vi "LV to ITX AutoPlot.vi"(0 "filename":string="filename", 1 "path":path=path "C:/", 5 "Notes":string, 7 "Data":cluster{"Y  Array":dbl[]}[](array[cluster]), 11 "wavenames (.Vx, etc)":string[](array[string])=["time", "x", "y", "z"], 12 "X,Y Labels":string[](array[string])=["x label", "y label"], 13 "X,Y Log":i32[](array[numeric])) -> (4 "file":path)   [LabVIEW 2013]
doc: "Write data to ITX file. This AutoPlot VI adds commands to automatically create a graph in Igor to quickly view your data.\n\n-- path: base path to save data\n-- filename: base filename\n-- Notes: add any notes here to help you remember what experiment you did\n-- Data: Cluster array\n It is recommended that you make the first cluster an array of timestamps\n-- wavenames: Give each data array a unique name such as \"time, bias, current,...\"zz\n-- X,Y Labels: For plotting in Igor. Can be ignored.\n-- X,Y Log: Do you wan to show X or Y on Log scale in Igor?"
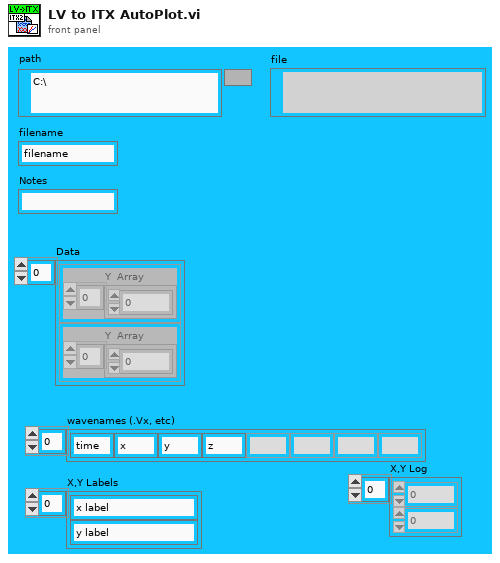
[diagram p1: front panel]
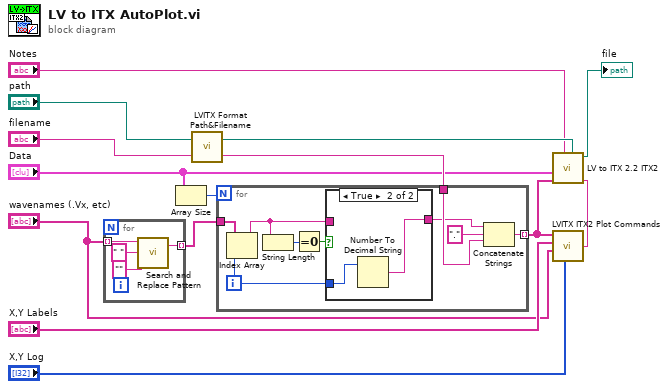
[diagram p0: block diagram]
diagram:
  n1 = for {
    tunnel: "wavenames (.Vx, etc)" -> [w16] mode=indexing
    tunnel: [w15] -> w1 mode=indexing
    n2 = call <vilib>:"Search and Replace Pattern.vi"("string"=w16, "regular expression (\"\")"=" " ("regular expression (\"\")"), "replace string (\"\")"="" ("replace string (\"\")")) -> ("result string"=w15:string)  [unwired: 2 in, 1 out]
  }
  n3 = Array Size(array="Data") -> (size(s)=w13:i32)
  n4 = call "LVITX Format Path&Filename.vi"("filename"="filename", "path"="path") -> ("file name without extension"=w12:string, "dup file"=w9:path)
  n5 = for {
    N: w13 -> [_]
    tunnel: w1 -> [w22]
    tunnel: w12 -> [w20]
    tunnel: [w27] -> w2 mode=indexing
    i -> [w23]
    n6 = Index Array(array=w22, index=w23) -> (element=w21:string)
    n7 = String Length(string=w21) -> (length=w24:i32)
    n8 = Equal To 0?(x=w24) -> (x = 0?=w25:bool)
    n9 = case shown="True" w25 {
      tunnel: w23 -> [_ w29]
      tunnel: [w28 w30] -> w19
      tunnel: w21 -> [w28 _]
      frame False {
      }
      frame True {
        n10 = Number To Decimal String(number=w29) -> (decimal integer string=w30:string)  [unwired: 1 out]
      }
    }
    n11 = Concatenate Strings(w19, "." ("string"), w20) -> (w27:string)
  }
  n12 = call "LVITX ITX2 Plot Commands.vi"("X,Y Log"="X,Y Log", "Plot labels"="wavenames (.Vx, etc)", "X,Y Labels"="X,Y Labels", "wavenames"=w2) -> ("result string"=w11:string)  [unwired: 2 in]
  n13 = call "LV to ITX 2.2 ITX2.vi"("Commands"=w11, "filename"=w9, "Notes"="Notes", "wavenames"=w2, "array of clusters"="Data") -> ("file"=→"file":path)  [unwired: 6 in]
